vi "Test Panel - Speciments (SubVI).vi"(8 "error in":errorcluster, 11 "Job ID":string) -> (0 "error out":errorcluster)   [LabVIEW 2019]
uses:
  Controls/Sample-state.ctl
  <vilib>/Utility/miscctls.llb/LVRowAndColumnTypeDef.ctl
  Controls/JSON - Sample.ctl
  <vilib>/httpClient/POSTBuffer.vi
  <vilib>/httpClient/LabVIEWHTTPClient.lvlib
panel:
  out "body":string
  in  "Remove":bool
  in  "Add":bool
  out "table specimen":string[][](table)
  in  "Close":bool
  in  "save":bool
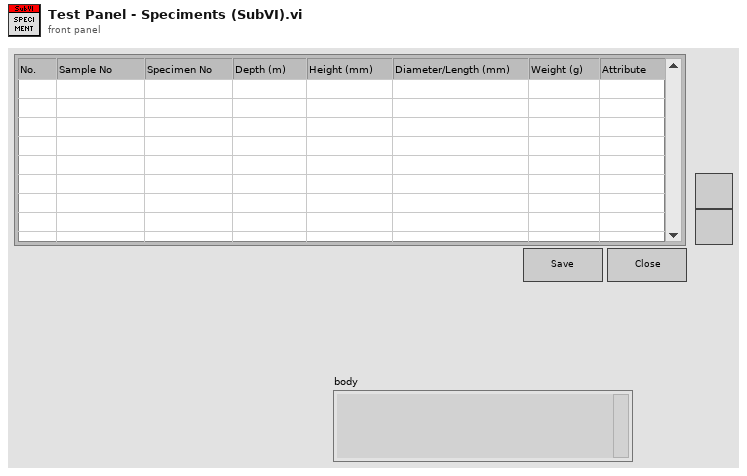
[diagram p1: front panel]
types:
  T1 = typedef "Sample-state.ctl" = enum16{"Init", "Read Config", "Idle", "Check", "Specimen", "Update", "Close"}
  T2 = typedef "LVRowAndColumnTypeDef.ctl" = cluster{"Row":i32, "Column":i32}
  T3 = cluster{"Key":string[], "Job No":string, "Job Desc":string, "Save":bool, "ID":string[], "No":string[], "Edit Position":T2}
  T4 = typedef "JSON - Sample.ctl" = cluster{"status":string, "data":cluster{"jobid":string, "sampleno":string, "specimentno":string, "weight":string, "height":string, "depth":string, "diameter":string, "delete":string, "id":string, "created_date":string, "attribute":string}[]}
  T5 = cluster{"action":string, "sampleno":string, "specimentno":string, "weight":string, "height":string, "depth":string, "diameter":string, "id":string, "jobid":string}
  T6 = cluster{"action":string, "jobid":string, "sampleno":string, "specimentno":string, "weight":string, "height":string, "depth":string, "diameter":string}
  T7 = cluster{"Jobs No":string, "Key Value":string[]}[]
  T8 = typedef "LabVIEWHTTPClient.lvlib/ClientHandle.ctl" = refnum<k1>
  T9 = cluster{"jobid":string, "sampleno":string, "specimentno":string, "weight":string, "height":string, "depth":string, "diameter":string, "delete":string, "id":string, "created_date":string, "attribute":string}[]
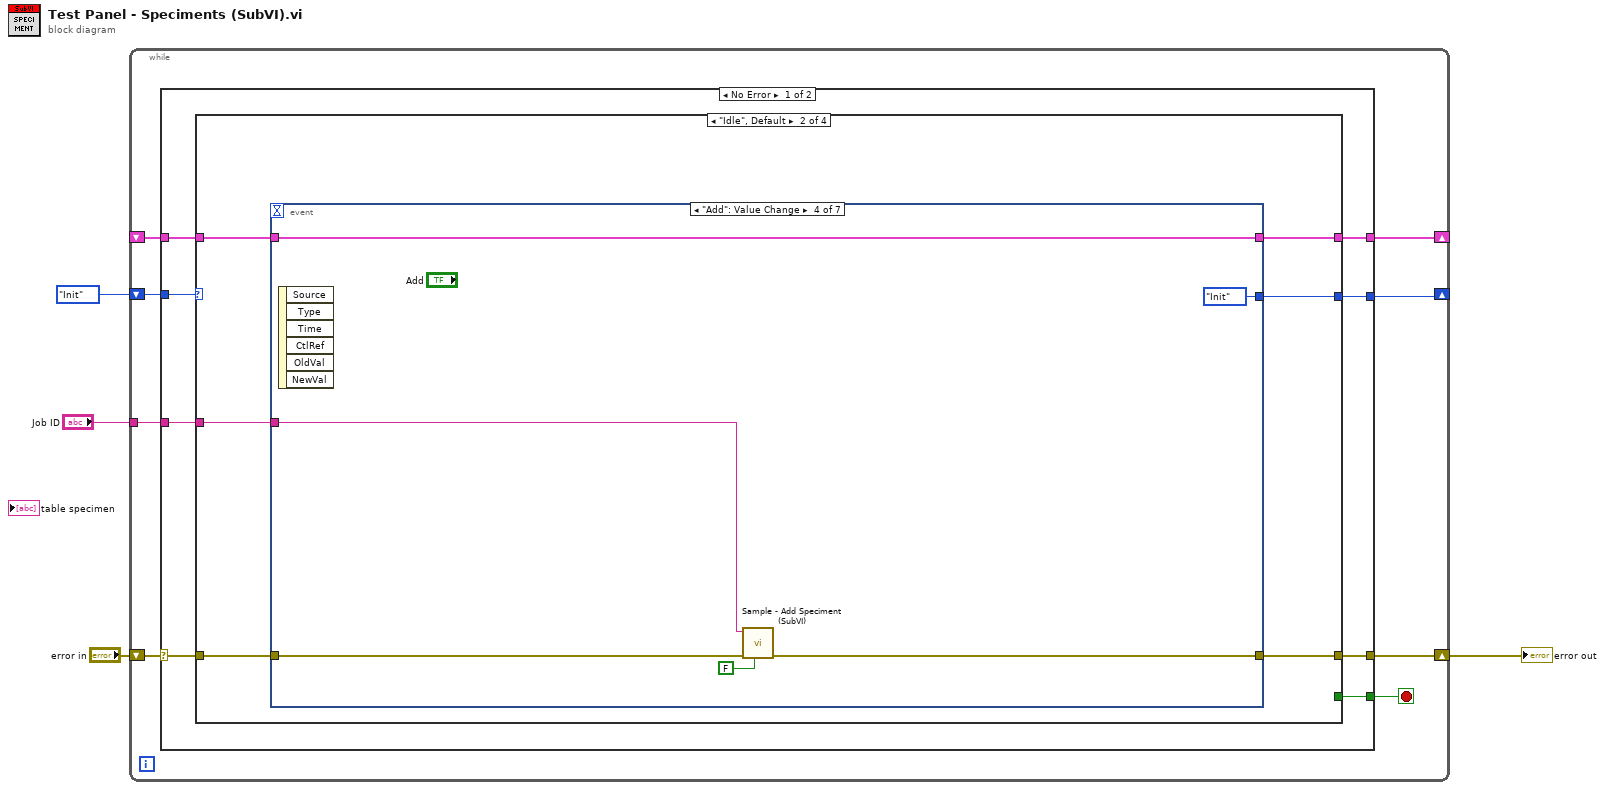
[diagram p0: block diagram]
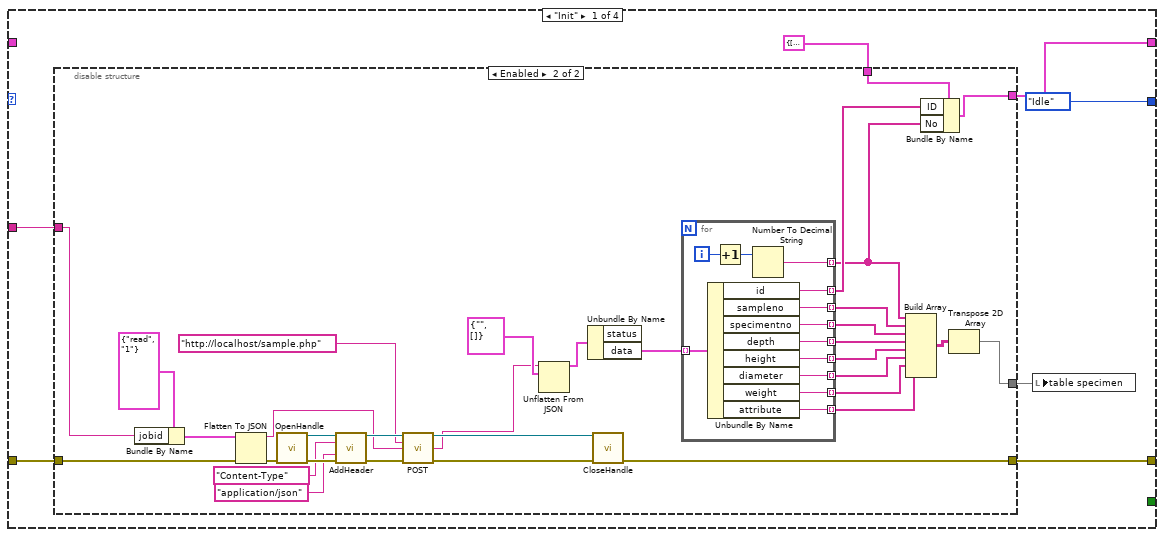
[diagram p2: hidden frame]
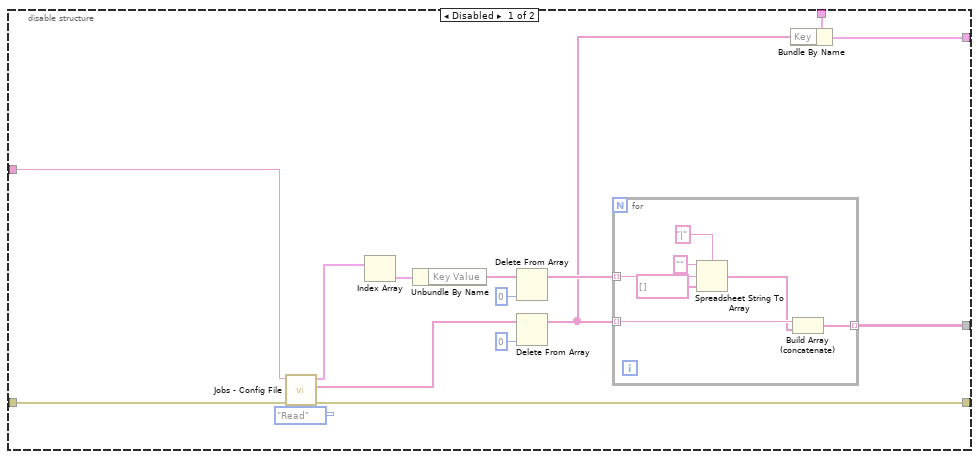
[diagram p3: hidden frame]
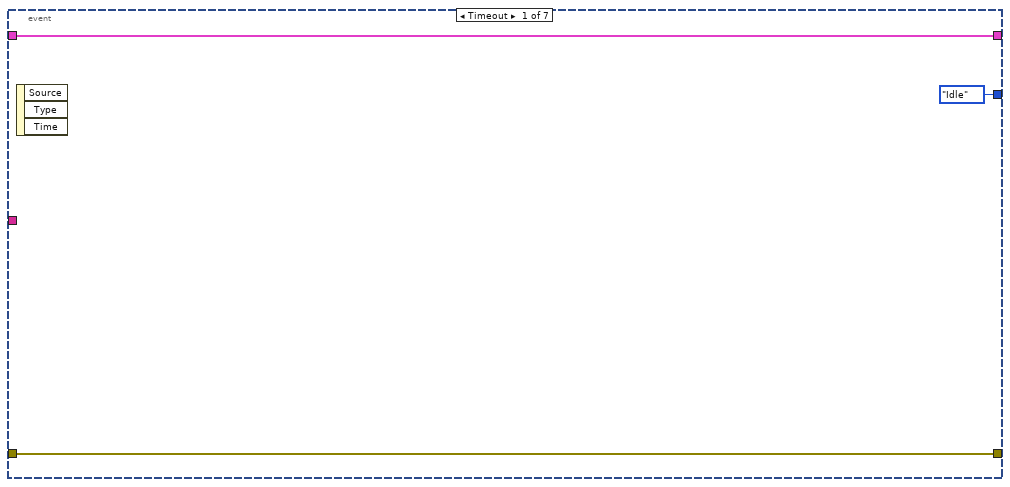
[diagram p4: hidden frame]
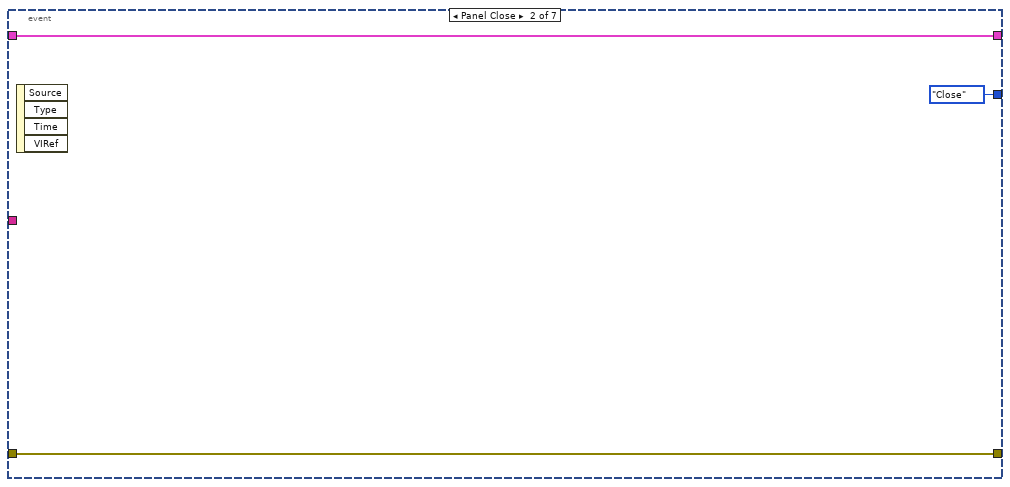
[diagram p5: hidden frame]
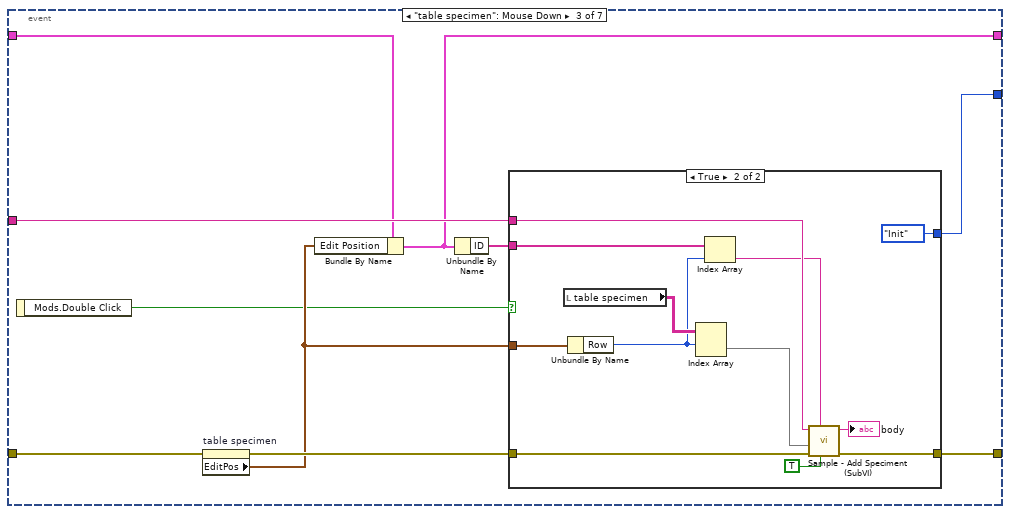
[diagram p6: hidden frame]
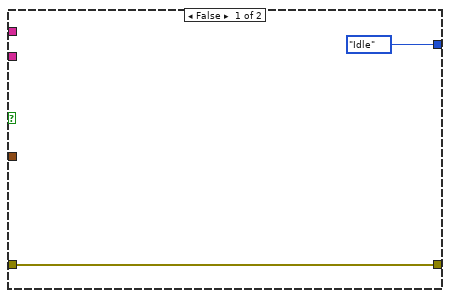
[diagram p7: hidden frame]
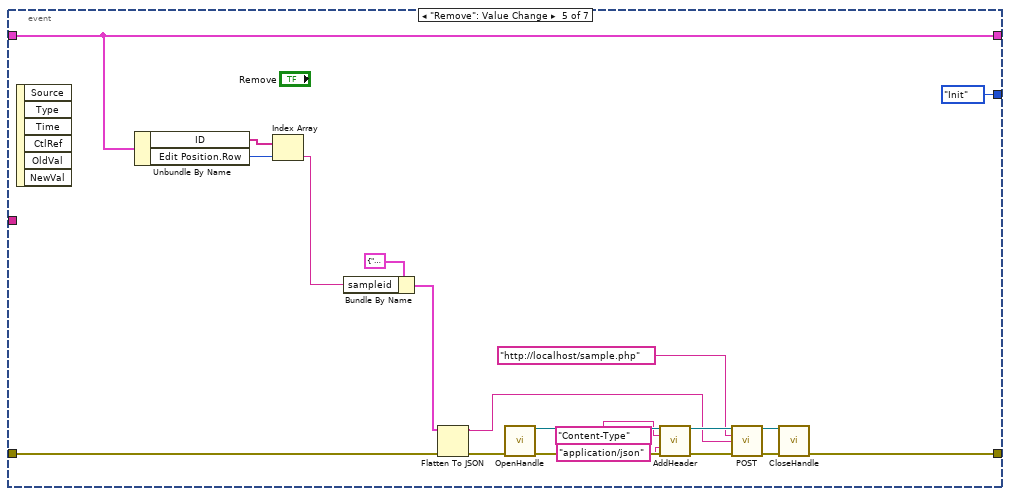
[diagram p8: hidden frame]
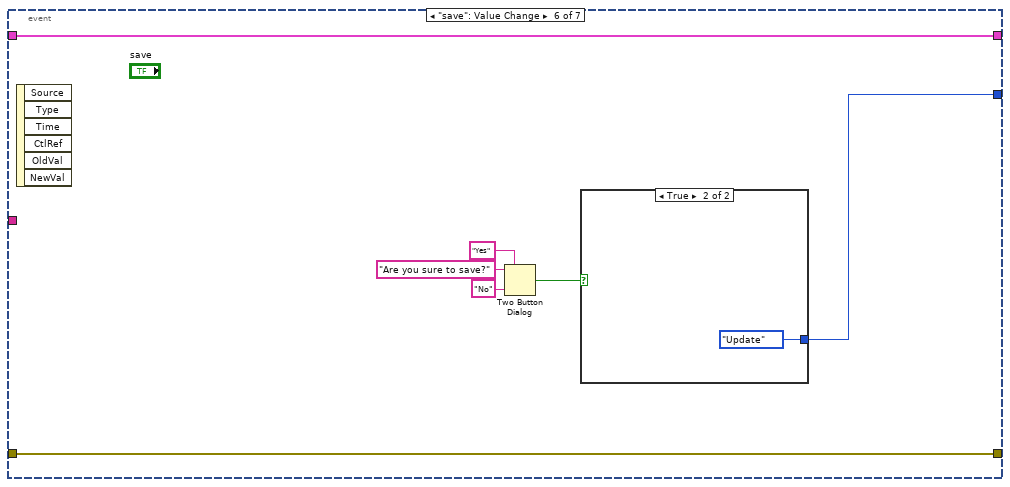
[diagram p9: hidden frame]
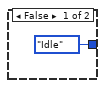
[diagram p10: hidden frame]
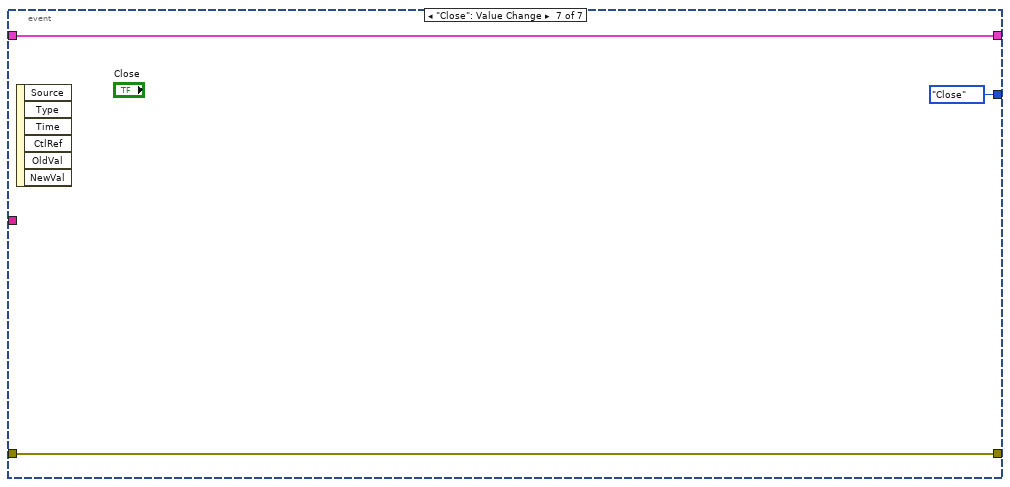
[diagram p11: hidden frame]
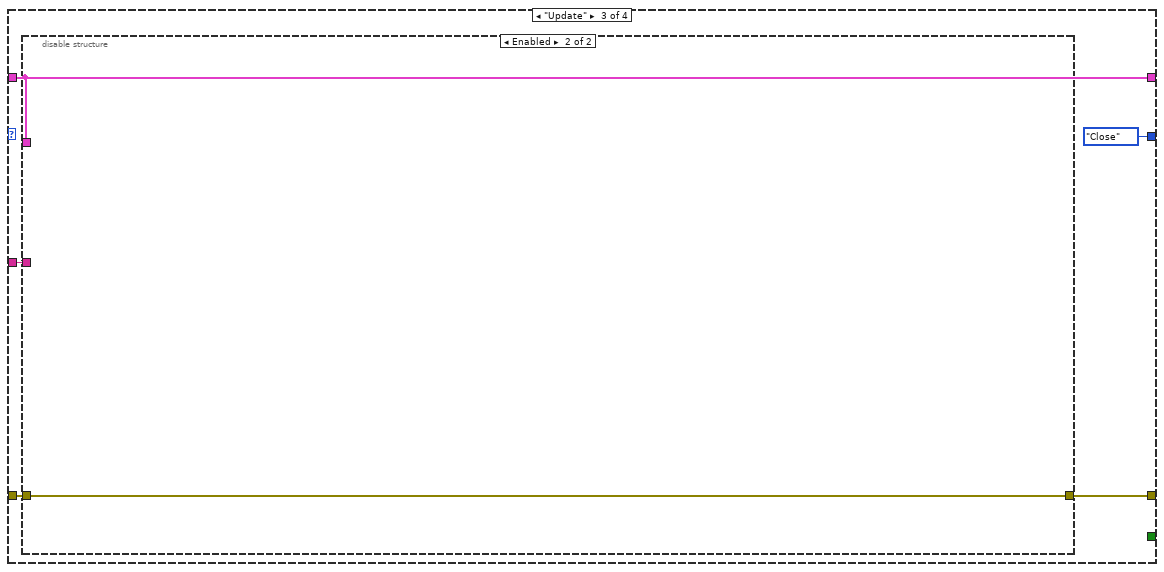
[diagram p12: hidden frame]
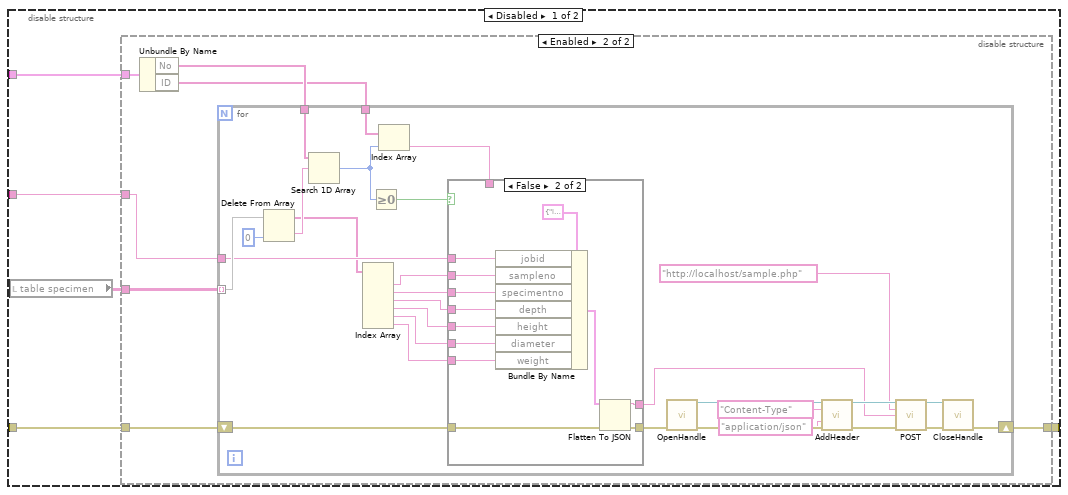
[diagram p13: hidden frame]
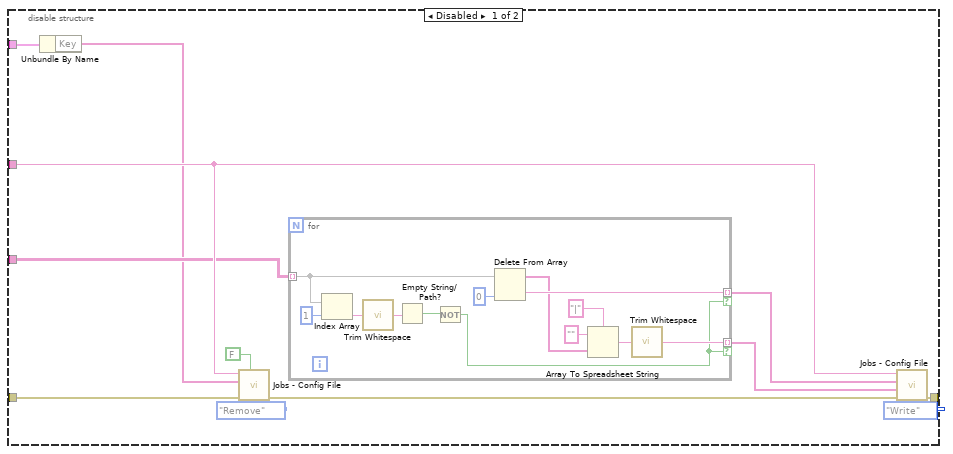
[diagram p14: hidden frame]
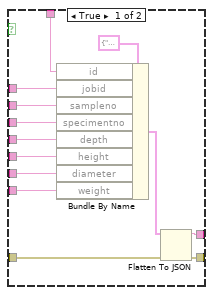
[diagram p15: hidden frame]
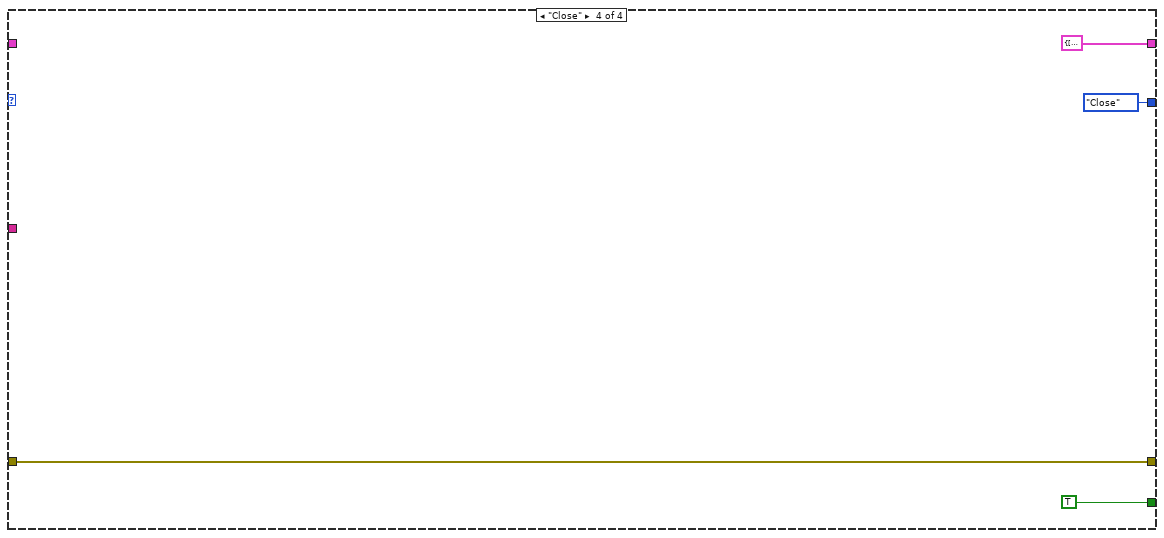
[diagram p16: hidden frame]
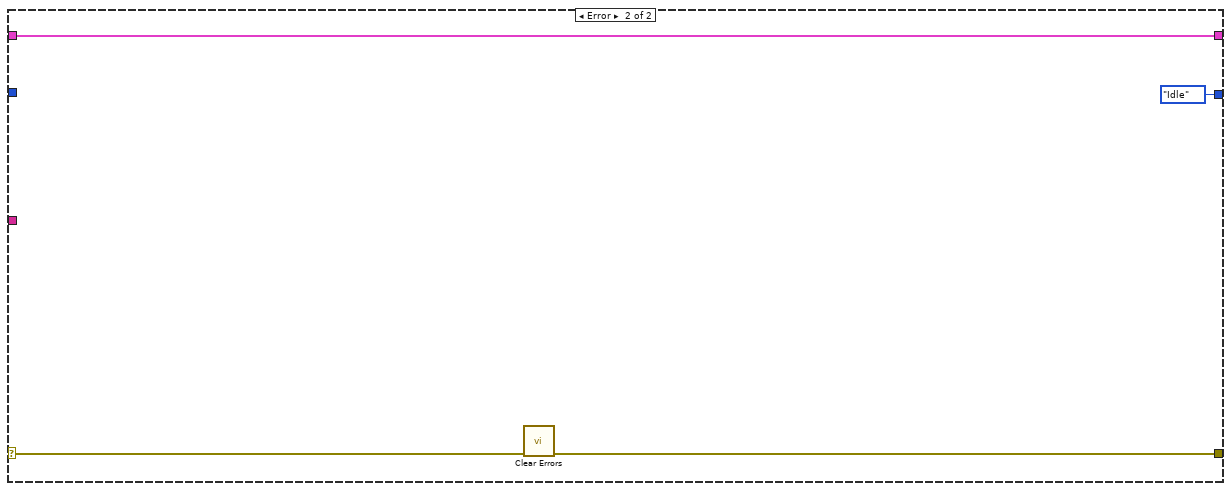
[diagram p17: hidden frame]
diagram:
  n1 = while {
    shift-right: [w10] -> w2
    shift-left: "error in" -> [w12]
    shift-right: [w9] -> _
    shift-left: Sample-state."Init" -> [w11]
    shift-right: [w8] -> _
    shift-left: _ -> [w7]
    tunnel: "Job ID" -> [w5]
    stop <- w6 stop-if-true
    n2 = case shown="No Error" w12 {
      selector: w12 -> [w19 w273]
      tunnel: w11 -> [w20 _]
      tunnel: [w18 w272] -> w10
      tunnel: [w17 Sample-state."Idle"] -> w9
      tunnel: [w16 w270] -> w8
      tunnel: w7 -> [w15 w270]
      tunnel: [w14 _] -> w6
      tunnel: w5 -> [w13 _]
      frame No Error {
        n3 = case shown="\"Idle\", Default" w20 {
          tunnel: w19 -> [w25 w100 w171 w268]
          tunnel: [w26 w99 w172 w268] -> w18
          tunnel: [Sample-state."Idle" w98 Sample-state."Close" Sample-state."Close"] -> w17
          tunnel: [w21 w96 w169 T3 {"Key"=[], "Job No"="", "Job Desc"="", "Save"=FALSE, "ID"=[], "No"=[], "Edit Position"={"Row"=0, "Column"=0}}] -> w16
          tunnel: w15 -> [_ w97 w169 _]
          tunnel: [_ _ _ TRUE] -> w14
          tunnel: w13 -> [w24 w95 w170 _]
          frame "Init" {
            n4 = disable-structure shown="Enabled" {
              disable-tunnel: [w41 w66] -> w26
              disable-tunnel: w25 -> [w40 w67]
              disable-tunnel: w24 -> [w39 w63]
              disable-tunnel: [w36 w55] -> w23
              disable-tunnel: T3 {"Key"=[], "Job No"="", "Job Desc"="", "Save"=FALSE, "ID"=[], "No"=[], "Edit Position"={"Row"=0, "Column"=0}} -> [w31 w54]
              disable-tunnel: [w30 w52] -> w21
              frame Disabled {
                n5 = call "Jobs - Config File.vi"("Action"=enum16{"Write", "Read", "Read All", "Remove"}."Read", "error in (no error)"=w40, "Jobs No"=w39) -> ("error out"=w41:errorcluster, "key names"=w29:string[], "Value Out"=w38:T7)  [unwired: 6 in]
                n6 = Index Array(array=w38) -> (element=w37:cluster{"Jobs No":string, "Key Value":string[]})  [unwired: 1 in]
                n7 = Unbundle By Name(w37) -> ("Key Value"=w34:string[])
                n8 = Delete From Array(array=w34, index=0) -> (array with subset deleted=w32:string[])  [unwired: 1 in, 1 out]
                n9 = Delete From Array(array=w29, index=0) -> (array with subset deleted=w28:string[])  [unwired: 1 in, 1 out]
                n10 = for {
                  tunnel: w28 -> [w45] mode=indexing
                  tunnel: w32 -> [w49] mode=indexing
                  tunnel: [w43] -> w36 mode=indexing
                  n11 = Spreadsheet String To Array(delimiter (Tab)="|", format string="", spreadsheet string=w49, array type (2D Dbl)=string[] []) -> (array=w44:string[])
                  n12 = Build Array (concatenate)(w45, w44) -> (w43:string[])
                }
                n13 = Bundle By Name(cluster=w31, "Key"=w28) -> (w30:T3)
              }
              frame Enabled {
                n14 = Bundle By Name(cluster=cluster{"action":string, "jobid":string} {"action"="read", "jobid"="1"}, "jobid"=w63) -> (w64:cluster{"action":string, "jobid":string})
                n15 = Flatten To JSON(anything=w64, error in (no error)=w67) -> (JSON string=w75:string, 11:w76:errorcluster)  [unwired: 1 in]
                n16 = call <vilib>:"OpenHandle.vi"("error in (no error)"=w76) -> ("client handle out"=w80:T8, "error out"=w82:errorcluster)  [unwired: 13 in]
                n17 = call <vilib>:"AddHeader.vi"("client handle"=w80, "header"="Content-Type", "value"="application/json", "error in (no error)"=w82) -> ("client handle out"=w79:T8, "error out"=w81:errorcluster)  [unwired: 10 in]
                n18 = call-poly <vilib>:"POST.vi"("client handle"=w79, "url"="http://localhost/sample.php", "buffer"=w75, "error in (no error)"=w81) -> ("client handle out"=w77:T8, "body"=w68:string, "error out"=w78:errorcluster)  [unwired: 8 in, 1 out]
                n19 = Unflatten From JSON(JSON string=w68, type and defaults=T4 {"status"="", "data"=[]}) -> (value=w70:T4)  [unwired: 5 in, 1 out]
                n20 = Unbundle By Name(w70) -> ("data"=w69:T9)  [unwired: 1 out]
                n21 = call <vilib>:"CloseHandle.vi"("client handle"=w77, "error in (no error)"=w78) -> ("error out"=w66:errorcluster)  [unwired: 13 in]
                n22 = for {
                  tunnel: w69 -> [w94] mode=indexing
                  tunnel: [w93] -> w62 mode=indexing
                  tunnel: [w92] -> w61 mode=indexing
                  tunnel: [w91] -> w60 mode=indexing
                  tunnel: [w88] -> w51 mode=indexing
                  tunnel: [w87] -> w59 mode=indexing
                  tunnel: [w86] -> w58 mode=indexing
                  tunnel: [w85] -> w57 mode=indexing
                  tunnel: [w84] -> w53 mode=indexing
                  tunnel: [w83] -> w50 mode=indexing
                  i -> [w90]
                  n23 = Unbundle By Name(w94) -> ("id"=w84:string, "sampleno"=w93:string, "specimentno"=w92:string, "depth"=w91:string, "height"=w87:string, "diameter"=w86:string, "weight"=w85:string, "attribute"=w83:string)
                  n24 = Increment(x=w90) -> (x+1=w89:i32)
                  n25 = Number To Decimal String(number=w89) -> (decimal integer string=w88:string)  [unwired: 1 in]
                }
                n26 = Build Array(w51, w62, w61, w60, w59, w58, w57, w50) -> (w56:string[][])
                n27 = Bundle By Name(cluster=w54, "ID"=w53, "No"=w51) -> (w52:T3)
                n28 = Transpose 2D Array(2D array=w56) -> (transposed array=w55:string[][])
              }
            }
            n29 = local write "table specimen"(w23) -> ()
          }
          frame "Idle", Default {
            n30 = event shown="[3] \"Add\": Value Change" {
              selector: _ -> [_ _ _ _ _ _ _]
              dyn-events: _ -> [_ _ _ _ _ _ _]
              timeout: _ -> [_ _ _ _ _ _ _]
              tunnel: w100 -> [w103 w106 w116 w133 w138 w161 w168]
              tunnel: [w103 w106 w114 w134 w139 w161 w168] -> w99
              tunnel: [Sample-state."Idle" Sample-state."Close" w107 Sample-state."Init" Sample-state."Init" w162 Sample-state."Close"] -> w98
              tunnel: w97 -> [w101 w105 w111 w136 w155 w160 w167]
              tunnel: [w101 w105 w108 w136 w155 w160 w167] -> w96
              tunnel: w95 -> [_ _ w113 w131 _ _ _]
              event Timeout {
                n31 = event-data() -> ()  [unwired: 1 in, 3 out]
              }
              event Panel Close {
                n32 = event-data() -> ()  [unwired: 1 in, 4 out]
              }
              event "table specimen": Mouse Down {
                n33 = event-data() -> ("Mods.Double Click"=w110:bool)  [unwired: 1 in]
                n34 = property on="table specimen" class="Tbl (strict)"(error in=w116) -> (error out=w115:errorcluster, "EditPos"=w112:T2)  [unwired: 1 in, 1 out]
                n35 = Bundle By Name(cluster=w111, "Edit Position"=w112) -> (w108:T3)
                n36 = Unbundle By Name(w108) -> ("ID"=w109:string[])
                n37 = case shown="True" w110 {
                  tunnel: w115 -> [w118 w129]
                  tunnel: [w118 w128] -> w114
                  tunnel: w113 -> [_ w127]
                  tunnel: w112 -> [_ w126]
                  tunnel: w109 -> [_ w121]
                  tunnel: [Sample-state."Idle" Sample-state."Init"] -> w107
                  frame False {
                  }
                  frame True {
                    n38 = local read "table specimen"() -> (w125:string[][])
                    n39 = Unbundle By Name(w126) -> ("Row"=w123:i32)
                    n40 = Index Array(array=w125, index (row)=w123) -> (element=w124:string[])  [unwired: 1 in]
                    n41 = Index Array(array=w121, index=w123) -> (element=w122:string)
                    n42 = call "Sample - Add Speciment (SubVI).vi"("Load?"=TRUE, "ID"=w122, "error in"=w129, "Data"=w124, "JobID"=w127) -> ("error in 2"=w128:errorcluster, "body"=→"body":string)  [unwired: 5 in]
                  }
                }
              }
              event "Add": Value Change {
                n43 = event-data() -> ()  [unwired: 1 in, 6 out]
                n44 = call "Sample - Add Speciment (SubVI).vi"("Load?"=FALSE, "error in"=w133, "JobID"=w131) -> ("error in 2"=w134:errorcluster)  [unwired: 7 in, 1 out]
              }
              event "Remove": Value Change {
                n45 = event-data() -> ()  [unwired: 1 in, 6 out]
                n46 = Unbundle By Name(w155) -> ("ID"=w154:string[], "Edit Position.Row"=w153:i32)
                n47 = Index Array(array=w154, index=w153) -> (element=w137:string)
                n48 = Bundle By Name(cluster=cluster{"action":string, "sampleid":string} {"action"="delete", "sampleid"=""}, "sampleid"=w137) -> (w143:cluster{"action":string, "sampleid":string})
                n49 = Flatten To JSON(anything=w143, error in (no error)=w138) -> (JSON string=w140:string, 11:w141:errorcluster)  [unwired: 1 in]
                n50 = call <vilib>:"OpenHandle.vi"("error in (no error)"=w141) -> ("client handle out"=w150:T8, "error out"=w152:errorcluster)  [unwired: 13 in]
                n51 = call <vilib>:"AddHeader.vi"("client handle"=w150, "header"="Content-Type", "value"="application/json", "error in (no error)"=w152) -> ("client handle out"=w149:T8, "error out"=w151:errorcluster)  [unwired: 10 in]
                n52 = call-poly <vilib>:"POST.vi"("client handle"=w149, "url"="http://localhost/sample.php", "buffer"=w140, "error in (no error)"=w151) -> ("client handle out"=w147:T8, "error out"=w148:errorcluster)  [unwired: 8 in, 2 out]
                n53 = call <vilib>:"CloseHandle.vi"("client handle"=w147, "error in (no error)"=w148) -> ("error out"=w139:errorcluster)  [unwired: 13 in]
              }
              event "save": Value Change {
                n54 = event-data() -> ()  [unwired: 1 in, 6 out]
                n55 = Two Button Dialog(message="Are you sure to save?", 1:"No" ("F button name (\"Cancel\")"), 2:"Yes" ("T button name (\"OK\")")) -> (T button?=w163:bool)
                n56 = case shown="True" w163 {
                  tunnel: [Sample-state."Idle" Sample-state."Update"] -> w162
                  frame False {
                  }
                  frame True {
                  }
                }
              }
              event "Close": Value Change {
                n57 = event-data() -> ()  [unwired: 1 in, 6 out]
              }
            }
          }
          frame "Update" {
            n58 = disable-structure shown="Enabled" {
              disable-tunnel: [w178 w265] -> w172
              disable-tunnel: w171 -> [w177 w265]
              disable-tunnel: w170 -> [w176 _]
              disable-tunnel: w169 -> [w175 _]
              frame Disabled {
                n59 = local read "table specimen"() -> (w174:string[][])
                n60 = disable-structure shown="Enabled" {
                  disable-tunnel: [w189 w205] -> w178
                  disable-tunnel: w177 -> [w184 w206]
                  disable-tunnel: w176 -> [w182 w204]
                  disable-tunnel: w174 -> [w181 w209]
                  disable-tunnel: w175 -> [w180 w210]
                  frame Disabled {
                    n61 = Unbundle By Name(w180) -> ("Key"=w179:string[])
                    n62 = call "Jobs - Config File.vi"("Action"=enum16{"Write", "Read", "Read All", "Remove"}."Remove", "Remove Section?"=FALSE, "error in (no error)"=w184, "Key Name"=w179, "Jobs No"=w182) -> ("error out"=w185:errorcluster)  [unwired: 4 in, 2 out]
                    n63 = for {
                      tunnel: w181 -> [w192] mode=indexing
                      tunnel: [w197] -> w187 mode=indexing if=w191
                      tunnel: [w199] -> w188 mode=indexing if=w191
                      n64 = Index Array(array=w192, index=1) -> (element=w193:string)
                      n65 = call <vilib>:"Trim Whitespace.vi"("string"=w193) -> ("trimmed string"=w194:string)  [unwired: 1 in]
                      n66 = Empty String/Path?(string/path=w194) -> (empty?=w195:bool)
                      n67 = Not(x=w195) -> (.not. x?=w191:bool)
                      n68 = Delete From Array(array=w192, index=0) -> (deleted portion=w199:string, array with subset deleted=w198:string[])  [unwired: 1 in]
                      n69 = Array To Spreadsheet String(delimiter (Tab)="|", array=w198, 3:"" ("format string")) -> (spreadsheet string=w201:string)
                      n70 = call <vilib>:"Trim Whitespace.vi"("string"=w201) -> ("trimmed string"=w197:string)  [unwired: 1 in]
                    }
                    n71 = call "Jobs - Config File.vi"("Action"=enum16{"Write", "Read", "Read All", "Remove"}."Write", "error in (no error)"=w185, "Value"=w187, "Key Name"=w188, "Jobs No"=w182) -> ("error out"=w189:errorcluster)  [unwired: 4 in, 2 out]
                  }
                  frame Enabled {
                    n72 = Unbundle By Name(w210) -> ("No"=w208:string[], "ID"=w207:string[])
                    n73 = for {
                      tunnel: w209 -> [w238] mode=indexing
                      tunnel: w208 -> [w237]
                      tunnel: w207 -> [w234]
                      shift-right: [w224] -> w205
                      shift-left: w206 -> [w219]
                      tunnel: w204 -> [w221]
                      n74 = Delete From Array(array=w238, index=0) -> (deleted portion=w236:string, array with subset deleted=w217:string[])  [unwired: 1 in]
                      n75 = Search 1D Array(1D array=w237, element=w236) -> (index of element=w235:i32)  [unwired: 1 in]
                      n76 = Index Array(array=w217) -> (element #1=w216:string, element #2=w215:string, element #3=w214:string, element #4=w213:string, element #5=w212:string, element #6=w211:string)  [unwired: 6 in]
                      n77 = Greater Or Equal To 0?(x=w235) -> (x >= 0?=w222:bool)
                      n78 = Index Array(array=w234, index=w235) -> (element=w223:string)
                      n79 = case shown="False" w222 {
                        tunnel: w223 -> [w252 _]
                        tunnel: w221 -> [w250 w264]
                        tunnel: [w248 w262] -> w220
                        tunnel: w219 -> [w247 w261]
                        tunnel: [w246 w260] -> w218
                        tunnel: w216 -> [w245 w258]
                        tunnel: w215 -> [w244 w257]
                        tunnel: w214 -> [w243 w256]
                        tunnel: w213 -> [w242 w255]
                        tunnel: w212 -> [w241 w254]
                        tunnel: w211 -> [w240 w253]
                        frame True {
                          n80 = Bundle By Name(cluster=T5 {"action"="update", "sampleno"="", "specimentno"="", "weight"="", "height"="", "depth"="", "diameter"="", "id"="", "jobid"=""}, "id"=w252, "jobid"=w250, "sampleno"=w245, "specimentno"=w244, "depth"=w243, "height"=w242, "diameter"=w241, "weight"=w240) -> (w249:T5)
                          n81 = Flatten To JSON(anything=w249, error in (no error)=w247) -> (JSON string=w248:string, 11:w246:errorcluster)  [unwired: 1 in]
                        }
                        frame False {
                          n82 = Bundle By Name(cluster=T6 {"action"="insert", "jobid"="", "sampleno"="", "specimentno"="", "weight"="", "height"="", "depth"="", "diameter"=""}, "jobid"=w264, "sampleno"=w258, "specimentno"=w257, "depth"=w256, "height"=w255, "diameter"=w254, "weight"=w253) -> (w263:T6)
                          n83 = Flatten To JSON(anything=w263, error in (no error)=w261) -> (JSON string=w262:string, 11:w260:errorcluster)  [unwired: 1 in]
                        }
                      }
                      n84 = call <vilib>:"OpenHandle.vi"("error in (no error)"=w218) -> ("client handle out"=w230:T8, "error out"=w228:errorcluster)  [unwired: 13 in]
                      n85 = call <vilib>:"AddHeader.vi"("client handle"=w230, "header"="Content-Type", "value"="application/json", "error in (no error)"=w228) -> ("client handle out"=w231:T8, "error out"=w229:errorcluster)  [unwired: 10 in]
                      n86 = call-poly <vilib>:"POST.vi"("client handle"=w231, "url"="http://localhost/sample.php", "buffer"=w220, "error in (no error)"=w229) -> ("client handle out"=w233:T8, "error out"=w232:errorcluster)  [unwired: 8 in, 2 out]
                      n87 = call <vilib>:"CloseHandle.vi"("client handle"=w233, "error in (no error)"=w232) -> ("error out"=w224:errorcluster)  [unwired: 13 in]
                    }
                  }
                }
              }
              frame Enabled {
              }
            }
          }
          frame "Close" {
          }
        }
      }
      frame Error {
        n88 = call <vilib>:"Clear Errors.vi"("error in (no error)"=w273) -> ("error out"=w272:errorcluster)  [unwired: 5 in, 1 out]
      }
    }
  }
  "error out" <- w2
